vi "tearDown.vi"(8 "error in (no error)":errorcluster, 11 "reference in":refnum<class "RT Start.lvclass">) -> (0 "error out":errorcluster, 3 "reference out":refnum<class "RT Start.lvclass">)   [LabVIEW 2016, in "RT Start.lvclass"]
doc: "tearDown runs after the test method has completed. Use this method to clean up any operations or references that were opened by setUp or the test method. Unit tests should be independent of other unit tests so this VI should ensure that the next test can run in a 'clean' test environment."
uses:
  RT Start.lvclass
  Utilities/Simulated FPGA/FPGA Sim.lvclass
  1553 Board/1553 Board.lvclass
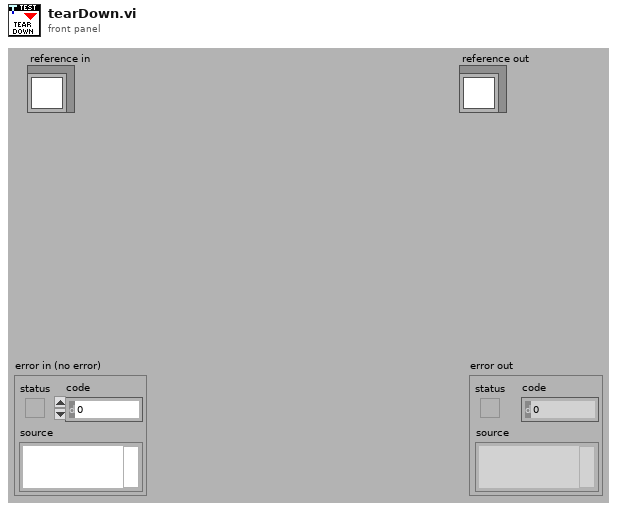
[diagram p1: front panel]
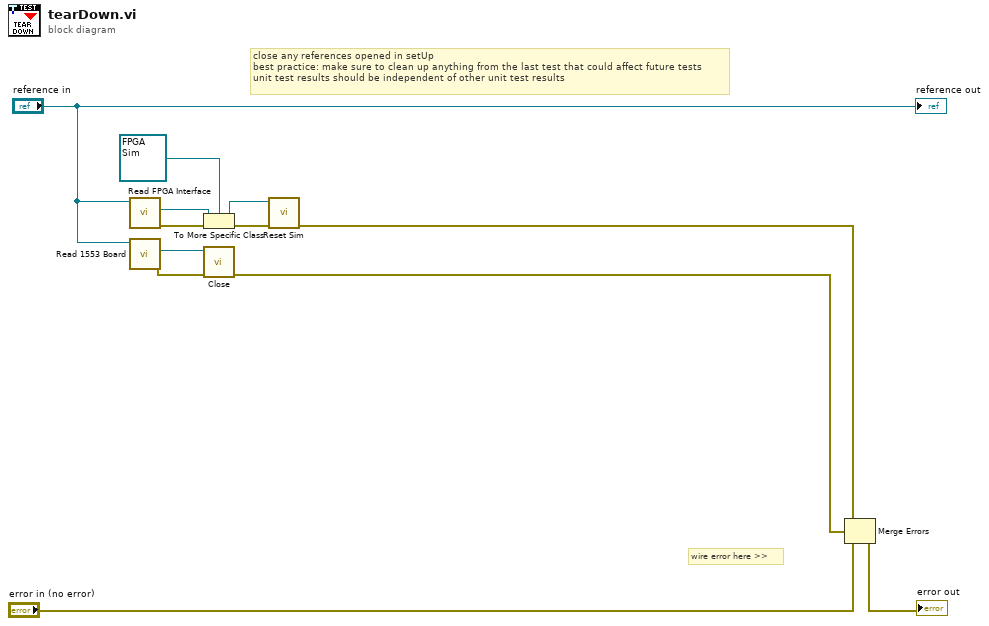
[diagram p0: block diagram]
diagram:
  # "wire error here >>"
  # "close any references opened in setUp\nbest practice: make sure to clean up anything from the last test that could affect future tests\nunit test results should be independent of other unit test results"
  n1 = call-dynamic "Read FPGA Interface.vi"("1553 Test in"="reference in") -> ("error out"=w5:errorcluster, "FPGA Interface"=w9:refnum<class "FPGA Interface.lvclass">)  [unwired: 8 in, 1 out]
  n2 = call-dynamic "Read 1553 Board.vi"("1553 Test in"="reference in") -> ("error out"=w6:errorcluster, "1553 Board"=w7:refnum<class "1553 Board.lvclass">)  [unwired: 8 in, 1 out]
  n3 = To More Specific Class(target class=refnum<class "FPGA Sim.lvclass"> refnum ("FPGA Sim.lvclass"), reference=w9, error in=w5) -> (specific class reference=w1:refnum<class "FPGA Sim.lvclass">, error out=w3:errorcluster)
  n4 = call-dynamic "Close.vi"("error in (no error)"=w6, "1553 Board in"=w7) -> ("error out"=w4:errorcluster)  [unwired: 9 in]
  n5 = call-dynamic "Reset Sim.vi"("error in (no error)"=w3, "FPGA Sim in"=w1) -> ("error out"=w2:errorcluster)  [unwired: 8 in, 1 out]
  n6 = Merge Errors(w2, w4, "error in (no error)") -> (→"error out":errorcluster)
  "reference out" <- "reference in"
